vi "calculate phi and Q.vi"() -> ()   [LabVIEW 2017]
panel:
  out "Q":dbl
  in  "Phi":dbl
  out "Phi":dbl
  in  "Length":dbl
  in  "amplitude":dbl
  in  "Q":dbl
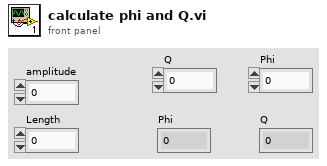
[diagram p1: front panel]
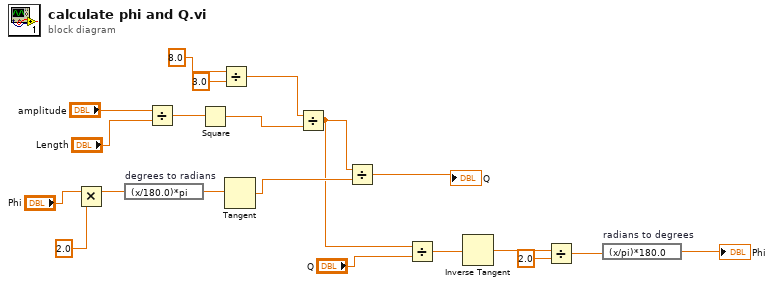
[diagram p0: block diagram]
diagram:
  n1 = Multiply(x="Phi", y=2.0) -> (x*y=w9:dbl)
  n2 = expression code="(x/180.0)*pi" "degrees to radians"(w9) -> (w12:dbl)
  n3 = Divide(x="amplitude", y="Length") -> (x/y=w18:dbl)
  n4 = Square(x=w18) -> (x^2=w14:dbl)
  n5 = Divide(x=8.0, y=3.0) -> (x/y=w15:dbl)
  n6 = Tangent(1:w12) -> (0:w11:dbl)
  n7 = Divide(x=w15, y=w14) -> (x/y=w7:dbl)
  n8 = Divide(x=w7, y=w11) -> (x/y=→"Q":dbl)
  n9 = Divide(x=w7, y="Q") -> (x/y=w5:dbl)
  n10 = Inverse Tangent(1:w5) -> (0:w4:dbl)
  n11 = Divide(x=w4, y=2.0) -> (x/y=w2:dbl)
  n12 = expression code="(x/pi)*180.0" "radians to degrees"(w2) -> (→"Phi":dbl)
